vi "create.ReduceSizeShort.vi"(8 "error in":errorcluster, 10 "ReduceSizeShort.Parameters":T1, 11 "ReduceSizeShort in":refnum<class "ReduceSizeShort.lvclass">) -> (0 "error out":errorcluster, 3 "ReduceSizeShort out":refnum<class "ReduceSizeShort.lvclass">)   [LabVIEW 2020, in "ReduceSizeShort.lvclass"]
uses:
  ReduceSizeShort.lvclass
  ReduceSizeShort.Parameters.ctl
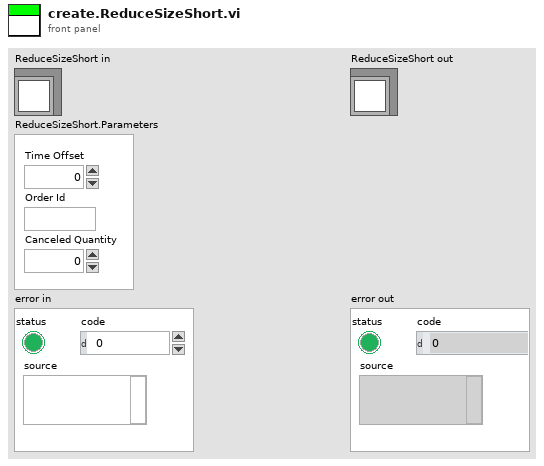
[diagram p1: front panel]
types:
  T1 = typedef "ReduceSizeShort.lvclass/ReduceSizeShort.Parameters.ctl" = cluster{"Time Offset":u32, "Order Id":string, "Canceled Quantity":u16}
  T2 = typedef "FieldSpec.ctl" = cluster{"Name":string, "Offset":i32, "Length":i32, "FieldType":enum16{"Alphanumeric", "Binary", "BinaryLongPrice", "BinaryShortPrice", "BitField", "PrintableAscii", "Value"}, "FieldValue":variant}
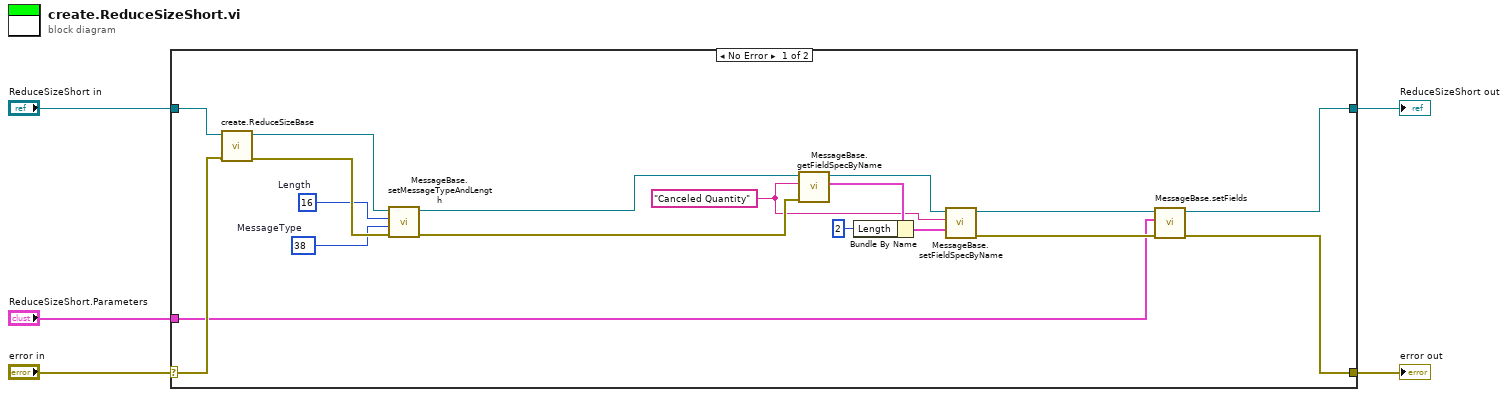
[diagram p0: block diagram]
diagram:
  n1 = case shown="No Error" "error in" {
    selector: "error in" -> [w11 w25]
    tunnel: [w6 w25] -> w4
    tunnel: [w7 w24] -> w2
    tunnel: "ReduceSizeShort in" -> [w12 w24]
    tunnel: "ReduceSizeShort.Parameters" -> [w8 _]
    frame No Error {
      w20 = u8 38  # MessageType
      w21 = u8 16  # Length
      w13 = "Canceled Quantity" ("Field.Name")
      n2 = call-dynamic "create.ReduceSizeBase.vi"("error in (no error)"=w11, "ReduceSizeBase in"=w12) -> ("error out"=w22:errorcluster, "ReduceSizeBase out"=w23:refnum<class "ReduceSizeShort.lvclass">)  [unwired: 8 in]
      n3 = call-dynamic "MessageBase.setMessageTypeAndLength.vi"("error in (no error)"=w22, "MessageType"=w20, "Length"=w21, "MessageBase in"=w23) -> ("error out"=w19:errorcluster, "MessageBase out"=w18:refnum<class "ReduceSizeShort.lvclass">)  [unwired: 6 in]
      n4 = call-dynamic "MessageBase.getFieldSpecByName.vi"("error in (no error)"=w19, "Field.Name"=w13, "MessageBase in"=w18) -> ("FIeldSpec"=w16:T2, "MessageBase out"=w17:refnum<class "ReduceSizeShort.lvclass">)  [unwired: 6 in, 1 out]
      n5 = Bundle By Name(cluster=w16, "Length"=2) -> (w14:T2)
      n6 = call-dynamic "MessageBase.setFieldSpecByName.vi"("FIeldSpec"=w14, "Field.Name"=w13, "MessageBase in"=w17) -> ("error out"=w9:errorcluster, "MessageBase out"=w10:refnum<class "ReduceSizeShort.lvclass">)  [unwired: 7 in]
      n7 = call-dynamic "MessageBase.setFields.vi"("error in (no error)"=w9, "Cluster (dup)"=w8, "MessageBase in"=w10) -> ("error out"=w6:errorcluster, "MessageBase out"=w7:refnum<class "ReduceSizeShort.lvclass">)  [unwired: 7 in]
    }
    frame Error {
    }
  }
  "error out" <- w4
  "ReduceSizeShort out" <- w2
